vi "Left regions to subsectors.vi"(1 "Left Regions":bool[](array[boolean])) -> (0 "Left subsector array":bool[][](array[boolean]))   [LabVIEW 2009]
doc: "Converts the marked regions to\ntwo dimensional arrays. Each \nelement in such an array is an\narray of marked regions for a \nparticular 18 degree wedge of\nthe sick's field of view, called a\n\"subector\"."
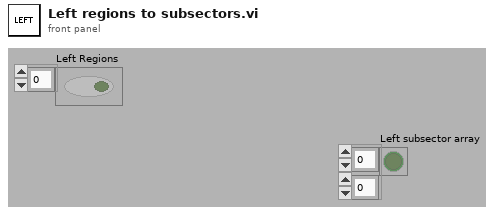
[diagram p1: front panel]
types:
  T1 = cluster{"Left Regions [0]":bool, "Left Regions [1]":bool, "Left Regions [2]":bool, "Left Regions [3]":bool, "Left Regions [4]":bool, "Left Regions [5]":bool, "Left Regions [6]":bool, "Left Regions [7]":bool, "Left Regions [8]":bool, "Left Regions [9]":bool, "Left Regions [10]":bool, "Left Regions [11]":bool, "Left Regions [12]":bool, "Left Regions [13]":bool, "Left Regions [14]":bool, "Left Regions [15]":bool, "Left Regions [16]":bool, "Left Regions [17]":bool, "Left Regions [18]":bool}
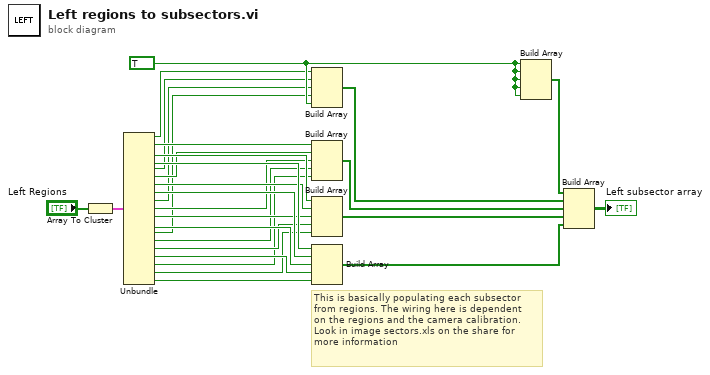
[diagram p0: block diagram]
diagram:
  w27 = TRUE
  # "This is basically populating each subsector\nfrom regions. The wiring here is dependent\non the regions and the camera calibration.\nLook in image sectors.xls on the share for\nmore information"
  n1 = Array To Cluster(array="Left Regions") -> (cluster=w28:T1)
  n2 = Unbundle(w28) -> ("Left Regions [0]"=w26:bool, "Left Regions [1]"=w25:bool, "Left Regions [2]"=w24:bool, "Left Regions [3]"=w23:bool, "Left Regions [4]"=w22:bool, "Left Regions [5]"=w21:bool, "Left Regions [6]"=w20:bool, "Left Regions [7]"=w19:bool, "Left Regions [8]"=w18:bool, "Left Regions [9]"=w17:bool, "Left Regions [10]"=w16:bool, "Left Regions [11]"=w15:bool, "Left Regions [12]"=w14:bool, "Left Regions [13]"=w13:bool, "Left Regions [14]"=w12:bool, "Left Regions [15]"=w11:bool, "Left Regions [16]"=w10:bool, "Left Regions [17]"=w9:bool, "Left Regions [18]"=w8:bool)
  n3 = Build Array(w26, w22, w18, w14, w27) -> (w6:bool[])
  n4 = Build Array(w25, w21, w17, w13, w10) -> (w5:bool[])
  n5 = Build Array(w24, w20, w16, w12, w9) -> (w4:bool[])
  n6 = Build Array(w23, w19, w15, w11, w8) -> (w3:bool[])
  n7 = Build Array(w27, w27, w27, w27, w27) -> (w7:bool[])
  n8 = Build Array(w7, w6, w5, w4, w3) -> (→"Left subsector array":bool[][])
